vi "Read Config.vi"(8 "error in (no error)":errorcluster, 9 "Re-Init?":bool, 10 "ICM File In":path, 11 "Clock Time in":refnum<class "Clock Time.lvclass">) -> (0 "error out":errorcluster, 3 "Clock Time out":refnum<class "Clock Time.lvclass">)   [LabVIEW 2018, in "Clock Time.lvclass"]
doc: "Clock Time.lvclass:Read Config.vi\n\nThis VI reads the Clock Time Class parameters from the ICM configuration file.\n\nInstrument Communication Module Version 1.0\nAugust, 2017 Original Code Consulting David Thomson\n www.originalcode.com"
uses:
  Clock Time.lvclass
  Clock Time.lvclass/Clock Time.ctl
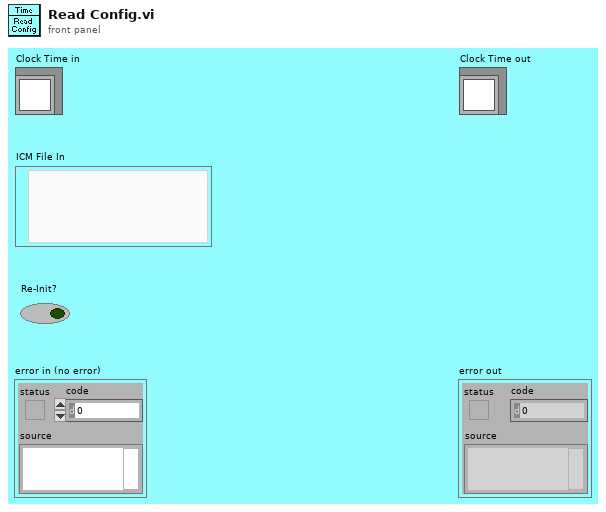
[diagram p1: front panel]
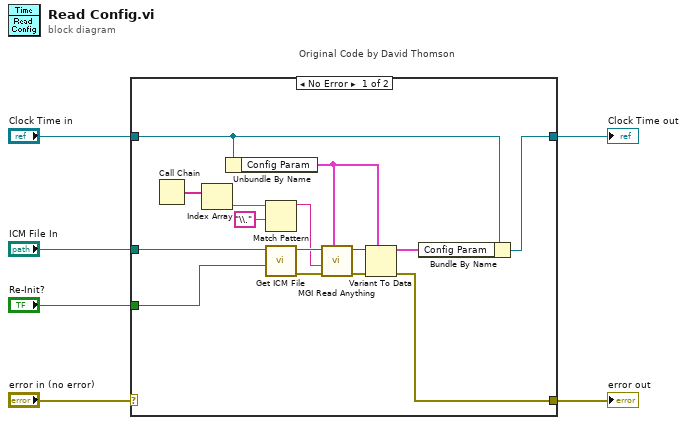
[diagram p0: block diagram]
diagram:
  n1 = case "Original Code by David Thomson" shown="No Error" "error in (no error)" {
    selector: "error in (no error)" -> [_ w23]
    tunnel: [w13 w23] -> w5
    tunnel: [w7 w22] -> w3
    tunnel: "Clock Time in" -> [w8 w22]
    tunnel: "ICM File In" -> [w10 _]
    tunnel: "Re-Init?" -> [w9 _]
    frame No Error {
      n2 = Call Chain() -> (call chain=w18:string[])
      n3 = Index Array(array=w18) -> (element=w19:string)  [unwired: 1 in]
      n4 = Unbundle By Name(w8) -> ("Config Param"=w11:cluster{"UTC?":bool})
      n5 = Match Pattern(string=w19, regular expression="\\.") -> (before substring=w16:string)  [unwired: 1 in, 3 out]
      n6 = call "Get ICM File.vi"("Re-Init?"=w9, "ICM File In"=w10) -> ("error out"=w20:errorcluster, "ICM File"=w21:path)  [unwired: 8 in]
      n7 = call <userlib>:"MGI Read Anything.vi"("Type of Anything"=w11, "Error In"=w20, "Section Name (Name of \"Type of Anything\")"=w16, "Path (dialog)"=w21) -> ("Error Out"=w14:errorcluster, "Anything"=w15:variant)  [unwired: 4 in, 2 out]
      n8 = Variant To Data(error in=w14, type=w11, Variant=w15) -> (data=w12:cluster{"UTC?":bool}, error out=w13:errorcluster)
      n9 = Bundle By Name(cluster=w8, "Config Param"=w12) -> (w7:refnum<class "Clock Time.lvclass">)
    }
    frame Error {
    }
  }
  "error out" <- w5
  "Clock Time out" <- w3
